vi "Configure Gating.vi"(6 "Enable Gating (F: Disable)":bool, 7 "Gating Type (0: BPASS)":i32(ring) items=["BPASS", "NOTCH"], 8 "error in (no error)":errorcluster, 9 "Gating Shape (2: Normal)":i32(ring)=2 items=["Maximum", "Wide", "Normal", "Minimum"], 10 "Channel (1)":i32=1, 11 "VISA resource name":refnum<visa-resource-name>) -> (0 "error out":errorcluster, 3 "VISA resource name out":refnum<visa-resource-name>)   [LabVIEW 2018, in "Keysight PNA Series.lvlib"]
doc: "Configures the gating filter."
uses:
  Keysight PNA Series.lvlib
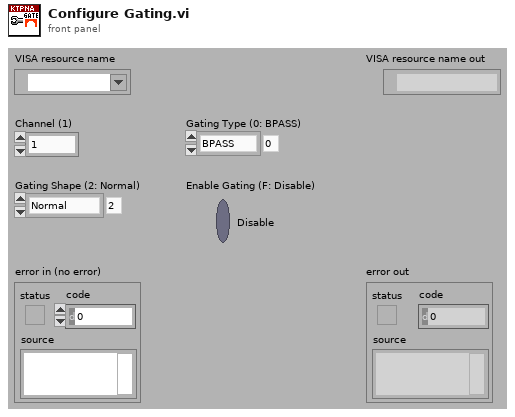
[diagram p1: front panel]
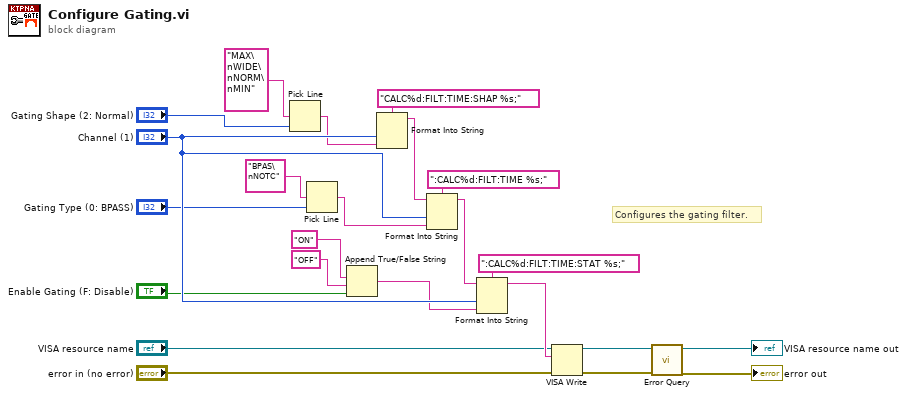
[diagram p0: block diagram]
diagram:
  # "Configures the gating filter."
  n1 = Pick Line(multi-line string="MAX\nWIDE\nNORM\nMIN", line index="Gating Shape (2: Normal)") -> (output string=w19:string)  [unwired: 1 in]
  n2 = Pick Line(multi-line string="BPAS\nNOTC", line index="Gating Type (0: BPASS)") -> (output string=w14:string)  [unwired: 1 in]
  n3 = Append True/False String(1:"Enable Gating (F: Disable)", 2:"OFF", 3:"ON") -> (0:w8:string)  [unwired: 1 in]
  n4 = Format Into String(format string="CALC%d:FILT:TIME:SHAP %s;", "Channel (1)", w19) -> (resulting string=w16:string)  [unwired: 2 in, 1 out]
  n5 = Format Into String(format string=":CALC%d:FILT:TIME %s;", initial string=w16, "Channel (1)", w14) -> (resulting string=w10:string)  [unwired: 1 in, 1 out]
  n6 = Format Into String(format string=":CALC%d:FILT:TIME:STAT %s;", initial string=w10, "Channel (1)", w8) -> (resulting string=w7:string)  [unwired: 1 in, 1 out]
  n7 = VISA Write(VISA resource name="VISA resource name", write buffer=w7, error in (no error)="error in (no error)") -> (VISA resource name out=w4:refnum<visa-resource-name>, error out=w3:errorcluster)  [unwired: 1 out]
  n8 = call "Error Query.vi"("error in (no error)"=w3, "VISA resource name"=w4) -> ("error out"=→"error out":errorcluster, "VISA resource name out"=→"VISA resource name out":refnum<visa-resource-name>)  [unwired: 6 in, 2 out]
